vi "Set Ring Text.vi"(6 "DIO ref":refnum<vi>, 10 "Inputs":string[](array[string]), 11 "Outputs":string[](array[string])) -> (4 "DIO ref out":refnum<vi>)   [LabVIEW 2015, in "Digital I-O.xctl"]
uses:
  Digital I-O.xctl
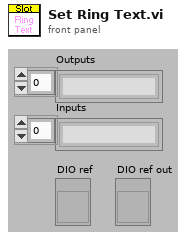
[diagram p1: front panel]
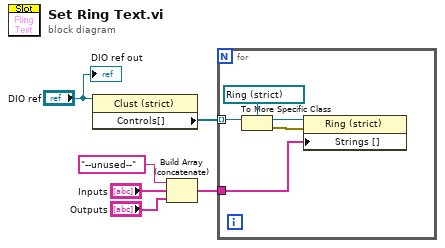
[diagram p0: block diagram]
diagram:
  n1 = property class="Clust (strict)"(reference="DIO ref") -> ("Controls[]"=w4:refnum<vi>[])  [unwired: 1 in, 2 out]
  n2 = Build Array (concatenate)("--unused--", "Inputs", "Outputs") -> (w6:string[])
  n3 = for {
    tunnel: w4 -> [w11] mode=indexing
    tunnel: w6 -> [w10]
    n4 = To More Specific Class(target class=refnum<vi> refnum ("Ring 2"), reference=w11) -> (specific class reference=w9:refnum<vi>, error out=w8:errorcluster)  [unwired: 1 in]
    n5 = property class="Ring (strict)"(reference=w9, error in=w8, "Strings []"=w10) -> ()  [unwired: 2 out]
  }
  "DIO ref out" <- "DIO ref"
